vi "CSM - Broadcast Console.vi"() -> ()   [LabVIEW 2017]
doc: "CSM Debug Console, you can use this tool:\n\n1. Select an existing CSM instance, open the front panel and block diagram.\n2. Scan the API interfaces of existing CSM instances.\n3. Select an API interface, call synchronously or asynchronously, view the return value.\n4. View the overall program's running log."
uses:
  _Support/Typedef/_CSM_List Module Scope.ctl
  _Support/Typedef/_CSM_GlobalLog_MSG.ctl
  _Support/Typedef/_CSM_Response Source Message.ctl
  _Support/Typedef/_CSM_GlobalLog_MSG_TYPE.ctl
  _jksm/_action.ctl
  1437127e-efa5-494e-aa43-da9d647a7a6f.vi
  6c6a0a0d-4e90-432b-9646-7a8ac0ceadb8.vi
  <vilib>/addons/_JKI Toolkits/State Machine/_JKI_lib_State_Machine.llb/Parse State Queue__JKI_lib_State_Machine.vi
  AdvanceAPI/CSM - Convert Error to Argument.vi
  _Support/GlobalEvent/GEvt-Generate with Rule Check.vi
  AdvanceAPI/CSM - Keywords.vi
  _Support/GlobalEvent/Cache-GEvt Refs.vi
  _Support/GlobalEvent/LogFilter/LogFilter - Check.vi
  <vilib>/Utility/Data Type/Get Type Information.vi
  _csmHelper/lvcsmFile/lvcsm File Path.vi
  <vilib>/Utility/config.llb/Open Config Data.vi
  <vilib>/Utility/config.llb/Read Key.vi
  <vilib>/Utility/config.llb/Read Key (Boolean).vi
  <vilib>/Utility/config.llb/Read Key (String).vi
  <vilib>/Utility/Data Type/Get Array Information.vi
  <vilib>/Utility/config.llb/Get Key Names.vi
  _csmHelper/lvcsmFile/Path to lvcsm String.vi
  _csmHelper/lvcsmFile/lvcsm String to Path.vi
  <vilib>/Utility/config.llb/Read Key (I32).vi
  <vilib>/Utility/config.llb/Read Key (Double).vi
  <vilib>/Utility/config.llb/Close Config Data.vi
  _csmHelper/lvcsmFile/_Array of VData to VCluster.vi
  <vilib>/Utility/config.llb/Write Key.vi
  <vilib>/Utility/config.llb/Write Key (Boolean).vi
  <vilib>/Utility/config.llb/Remove Key.vi
  <vilib>/Utility/config.llb/Write Key (String).vi
  <vilib>/Utility/config.llb/Write Key (I32).vi
  <vilib>/Utility/config.llb/Write Key (Double).vi
  _Polymophic/Build Synchronous Message with Arguments.vi
  _Polymophic/Build No-Reply Asynchronous Message with Arguments.vi
  _Polymophic/Build Interrupt Broadcast Message.vi
  _Support/GlobalEvent/LogFilter/LogFilter.lvclass
  Communicable State Machine.lvlib
  _csmHelper/API with lvcsm Support/CSM-Helper API with lvcsm Support.lvlib
  _csmHelper/CSM-Helper.lvclass
  _Shared/CSM Shared.lvlib
  _ui/csm-ui-support.lvlib
  _jksm/_jkism_magic.lvlib
panel:
  in  "Scope":T1
  in  "Refresh CSMs Button":bool
  in  "CSM":string(combo)
  in  "Interface-Filter":enum16{"API-Only", "UserDef States", "All"}(ring)
  in  "Refresh API":bool
  in  "MsgString":string(combo)
  in  "Tab(Msg/Status)":enum32{"Message", "Status"}(tab)
  in  "Sync (-@)":bool
  in  "Async (->|)":bool
  in  "Timeout(s)":i32=10 caption="(s)" min=1 max=180 step=1 format="%.0p"
  in  "Broadcast":bool
  in  "Arguments":string
  in  "Revert Safe String":bool=TRUE
  out "Response":string
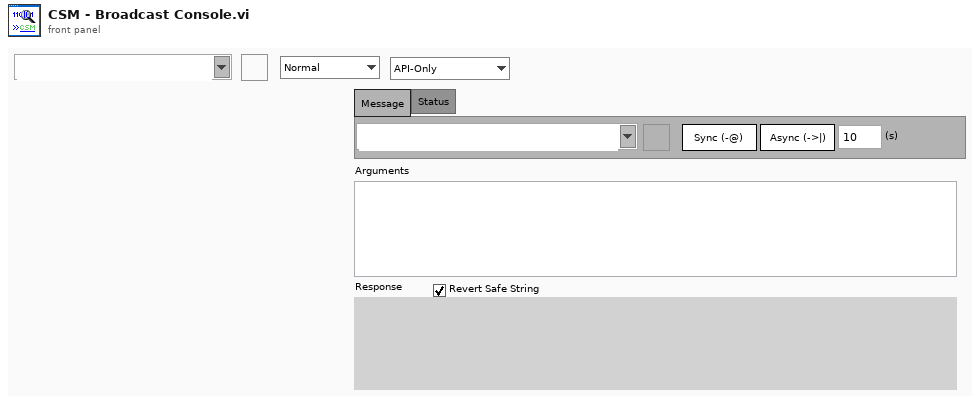
[diagram p1: front panel]
types:
  T1 = typedef "Communicable State Machine.lvlib/_CSM_List Module Scope.ctl" = enum16{"Normal", "System Only", "All"}
  T2 = enum32{"Invalid", "Standard", "Closed", "Hidden", "Minimized", "Maximized"}
  T3 = enum32{"invalid app kind", "Development System", "Run Time System", "Student Edition", "Embedded LabVIEW", "Evaluation", "Custom"}
  T4 = cluster{"Response Timeout(s)":i32, "History Length":i32, "History":string[], "Periodic Enable":bool, "Periodic threashold(#/s)":dbl, "Periodic Check Peroid(s)":dbl}
  T5 = typedef "_jkism_magic.lvlib/_action.ctl" = enum16{"Obtain", "Destroy", "Broadcast", "Post"}
  T6 = enum8{"Enabled", "Disabled", "Disabled and Grayed Out"}
  T7 = cluster{"Shift":bool, "Ctrl":bool, "Alt":bool, "Cmd":bool, "Opt":bool}
  T8 = cluster{"Core":cluster{"Current VI Reference":refnum<vi>, "Close Panel on Exit?":bool}, "CSM Global Log Event":refnum<user-event>, "MessageList":string[], "Toobar.advance":refnum<vi>[], "CSM Check History":string[], "History Length":i32}
  T9 = cluster{"Current VI Reference":refnum<vi>, "Close Panel on Exit?":bool}
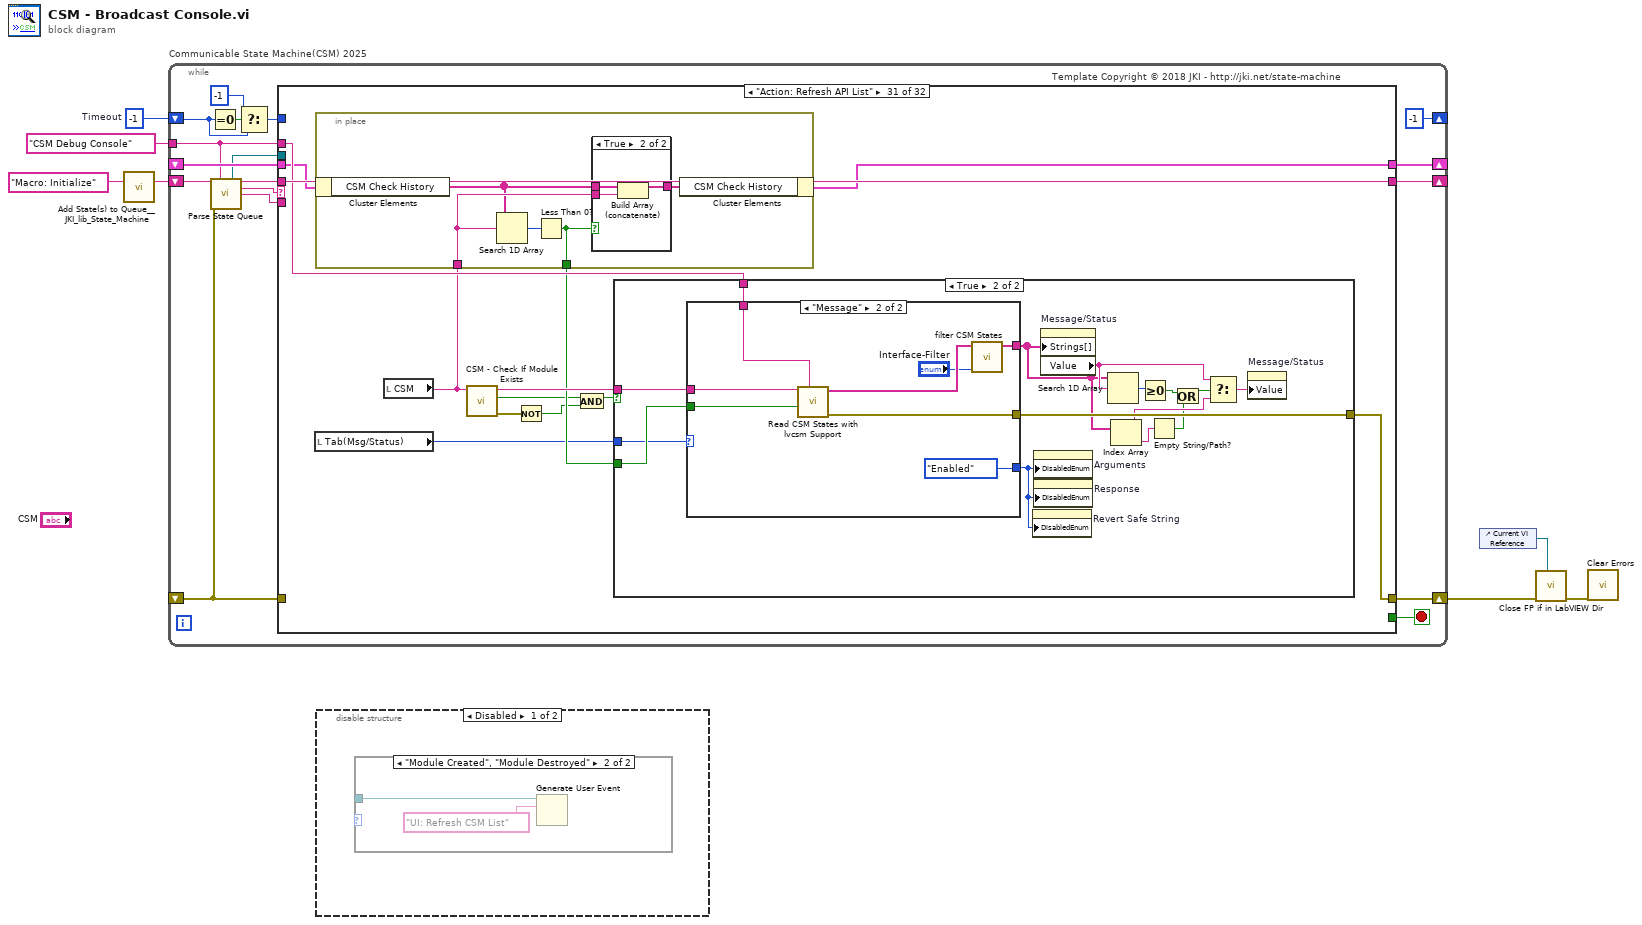
[diagram p0: block diagram]
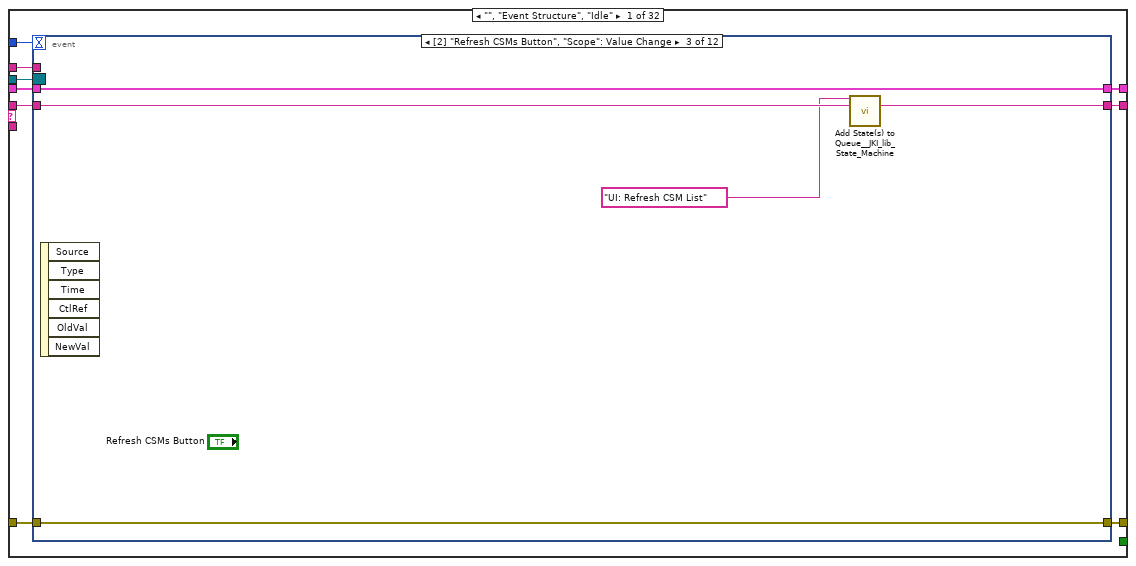
[diagram p4: hidden frame]
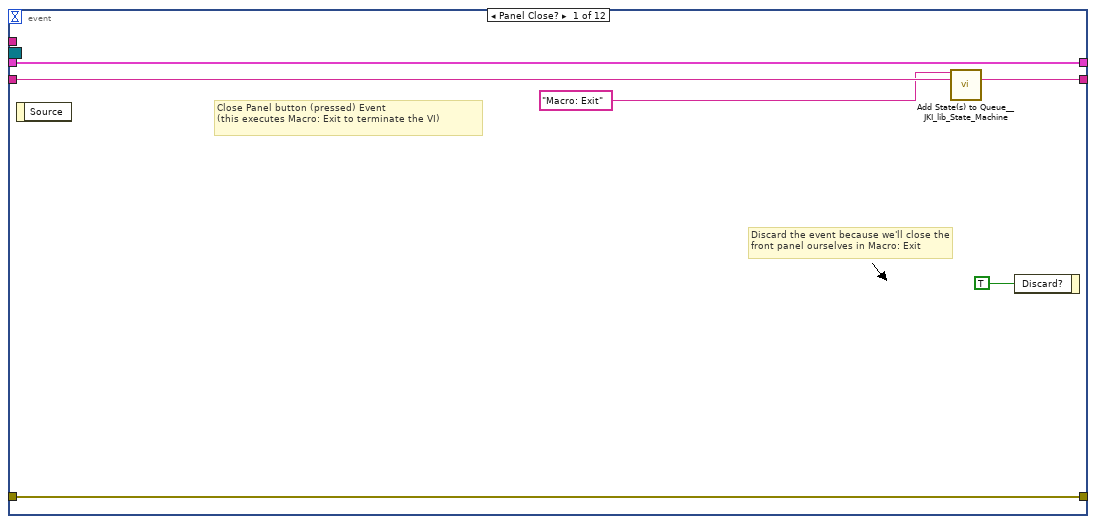
[diagram p5: hidden frame]
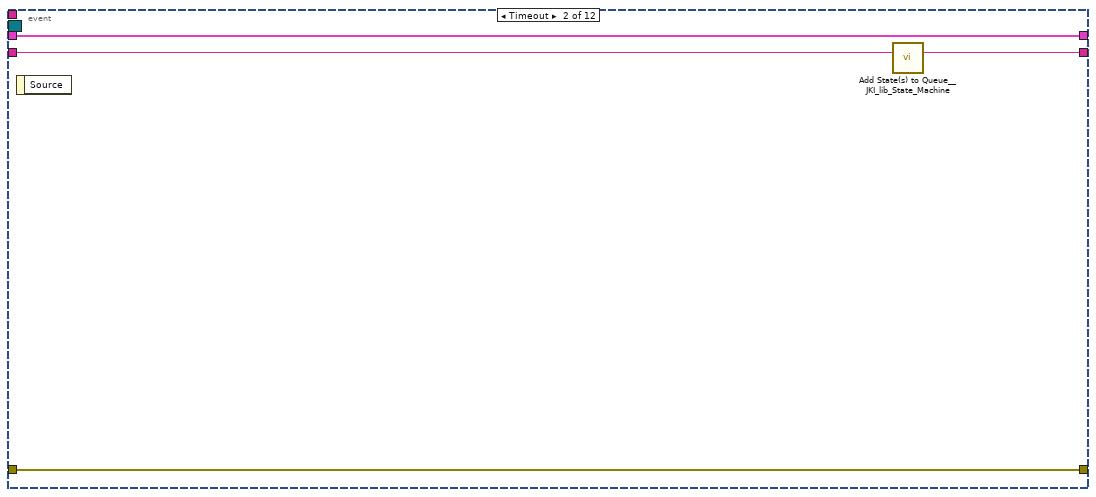
[diagram p6: hidden frame]
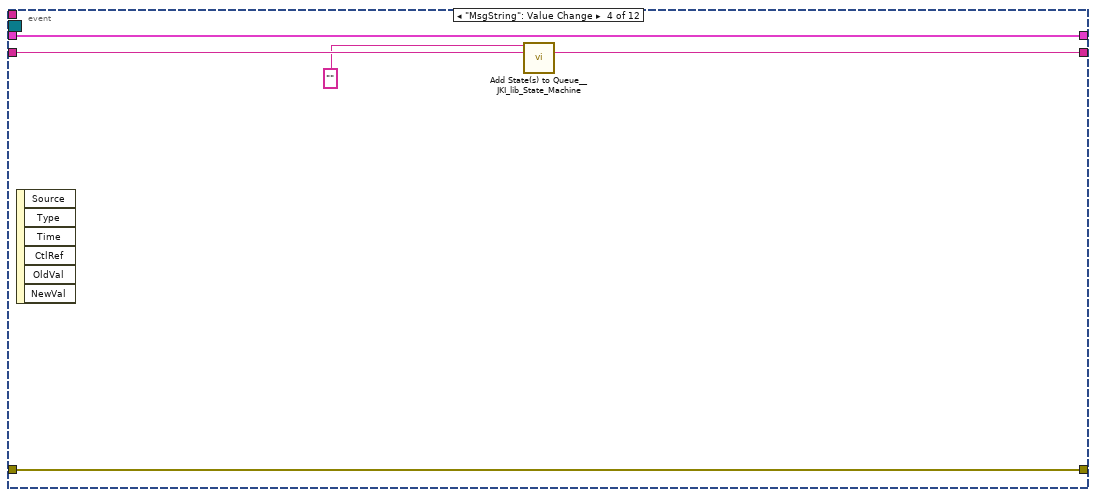
[diagram p7: hidden frame]
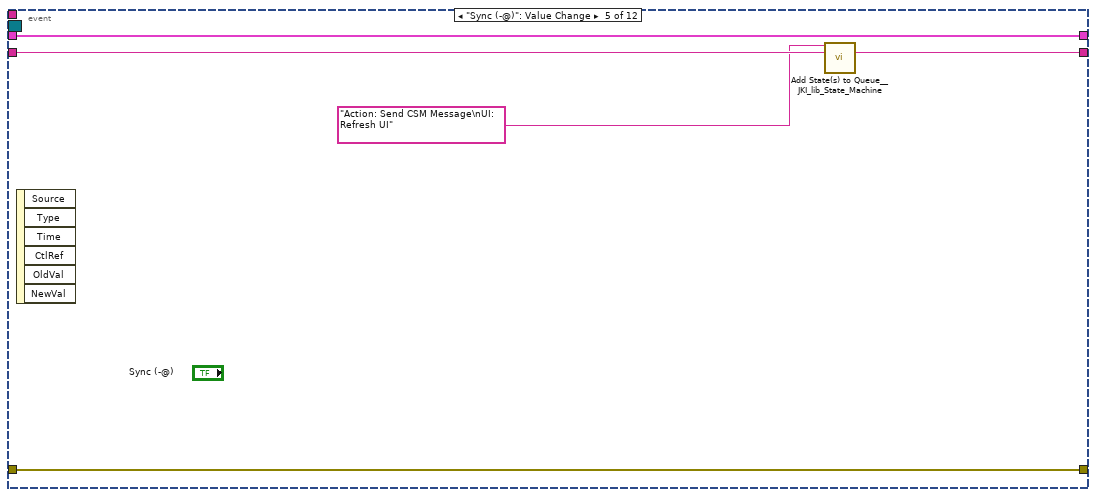
[diagram p8: hidden frame]
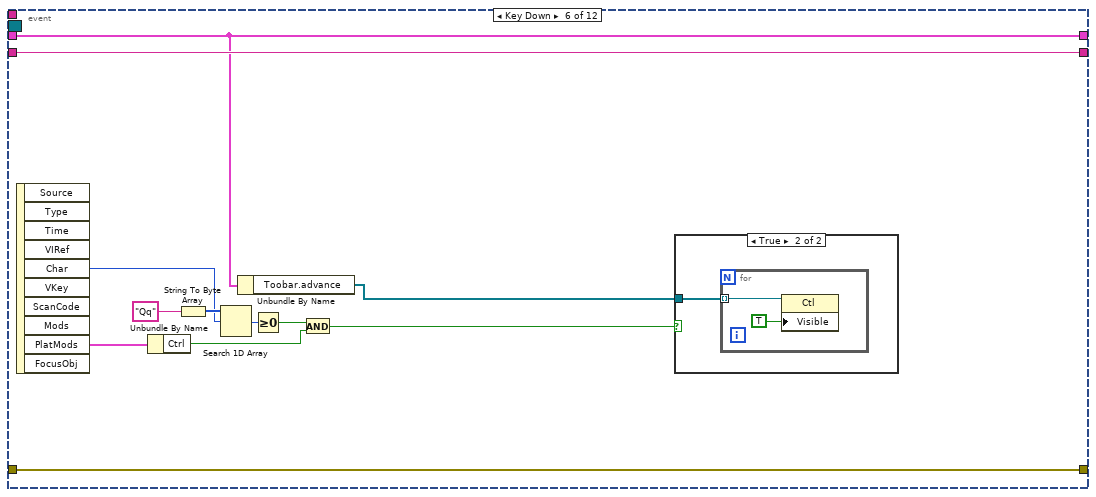
[diagram p9: hidden frame]
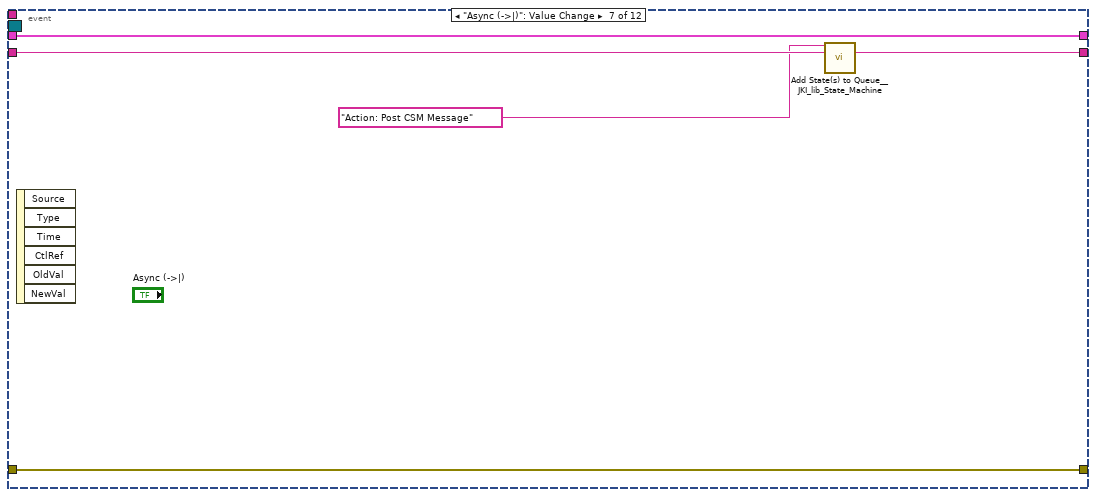
[diagram p11: hidden frame]
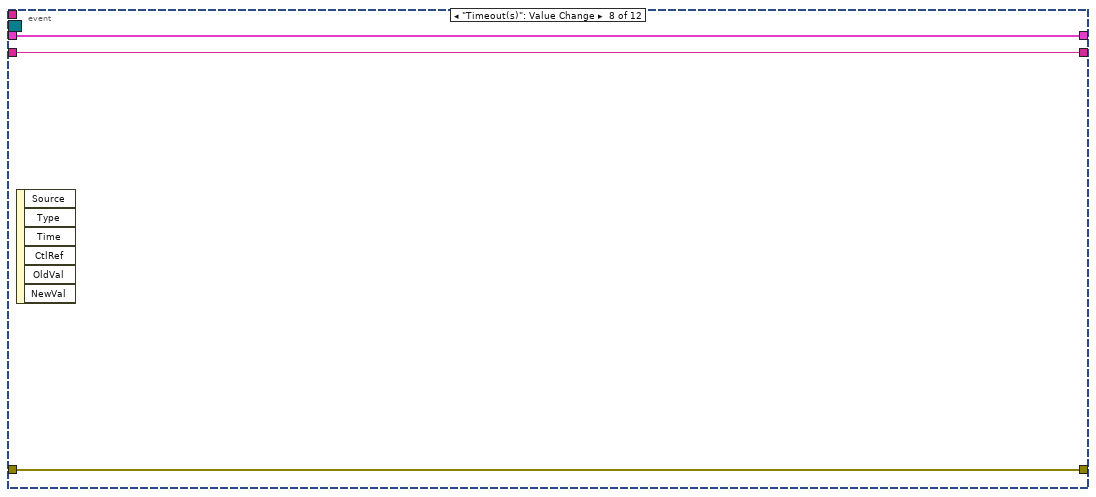
[diagram p12: hidden frame]
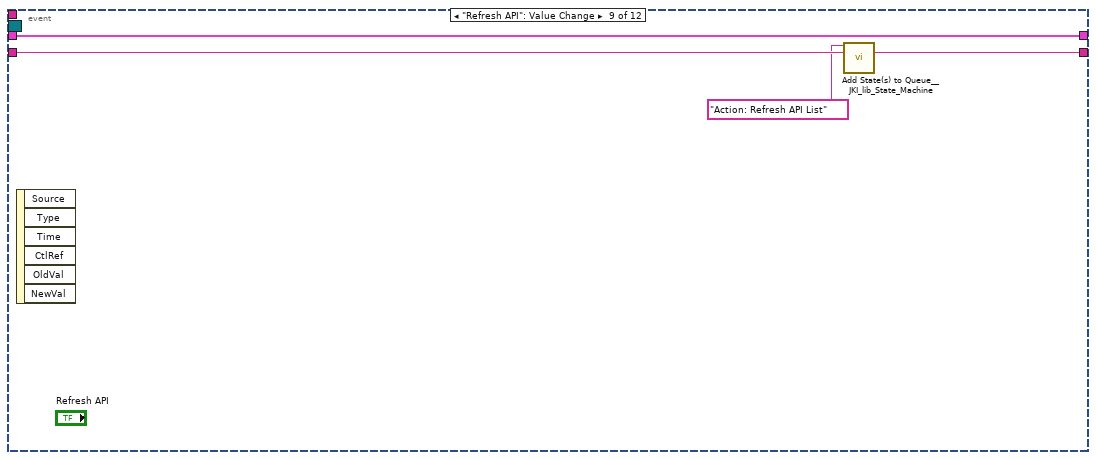
[diagram p13: hidden frame]
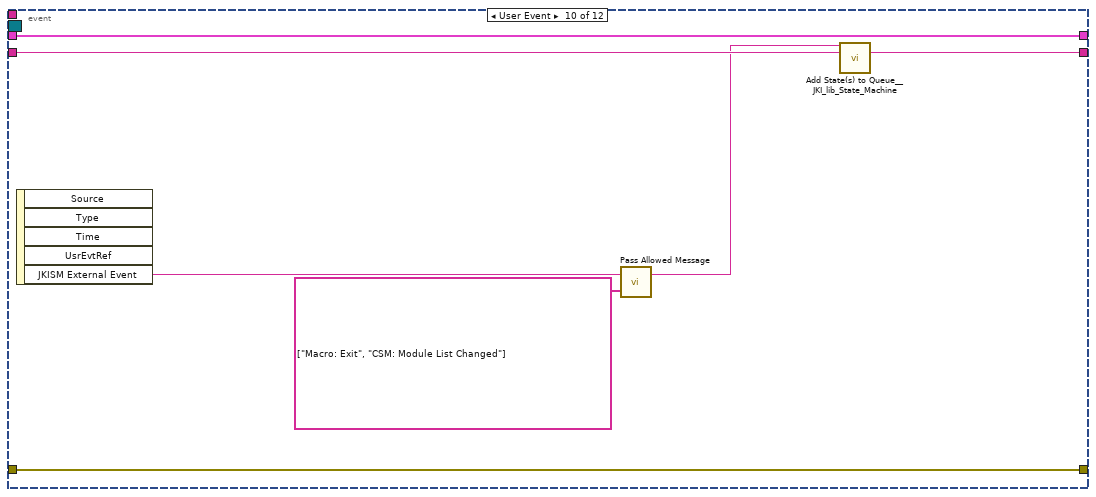
[diagram p14: hidden frame]
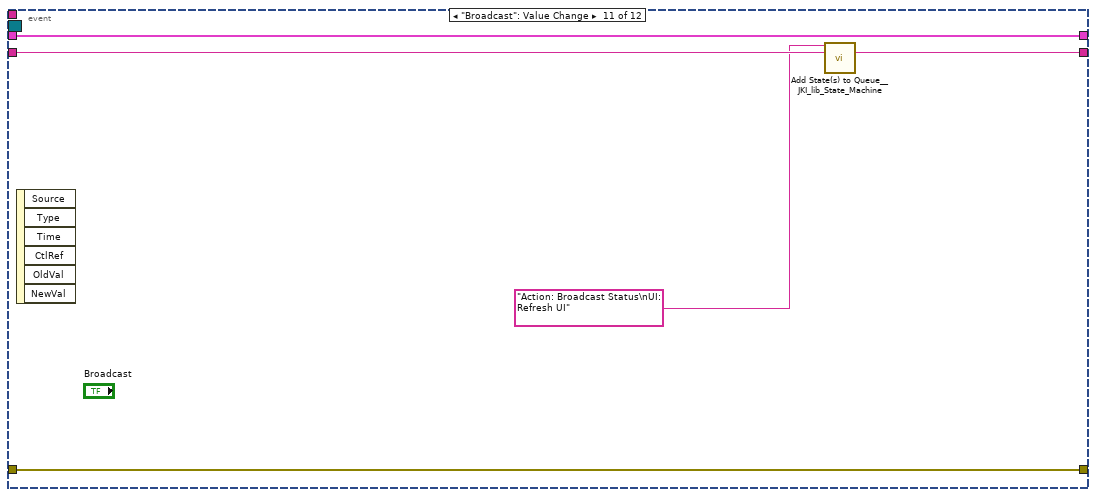
[diagram p15: hidden frame]
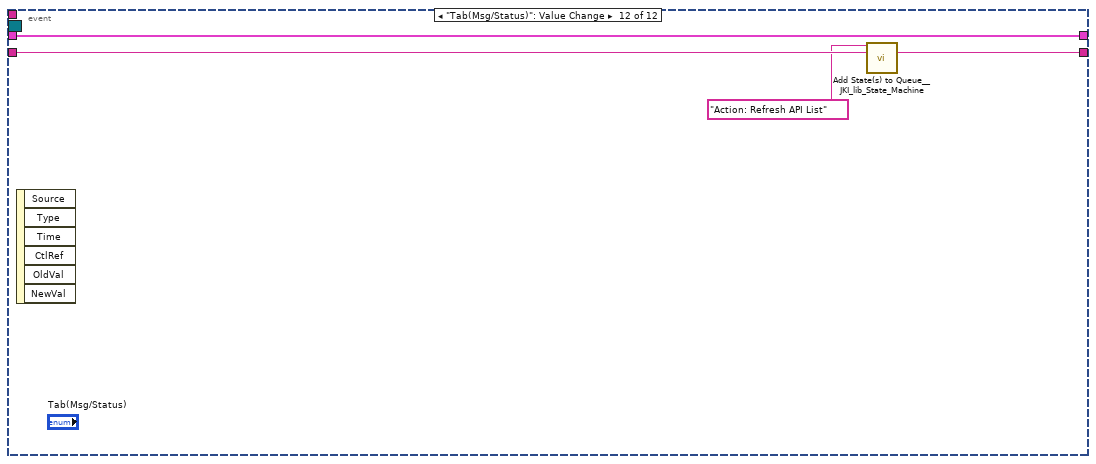
[diagram p16: hidden frame]
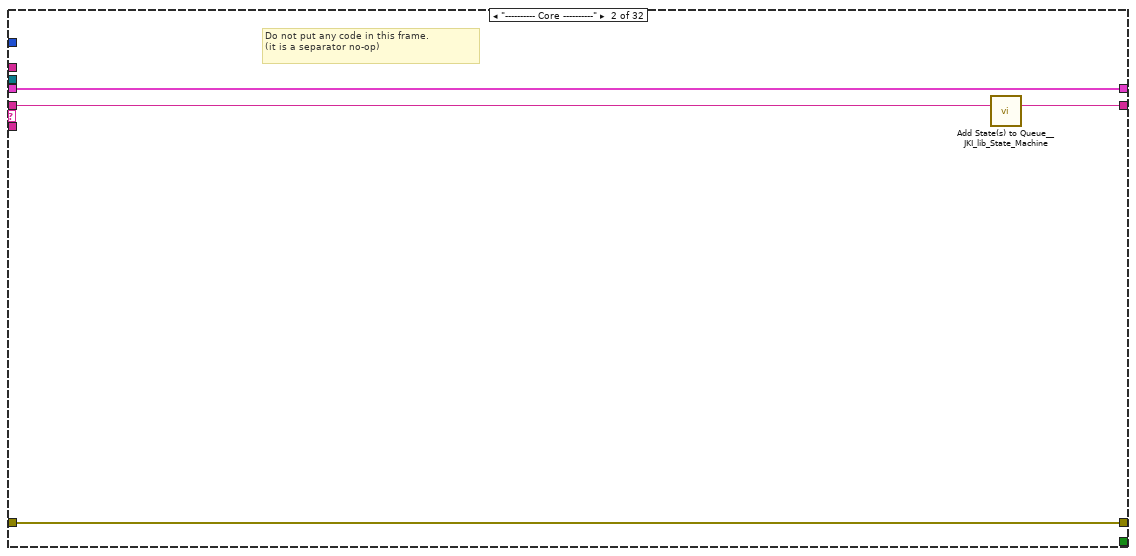
[diagram p17: hidden frame]
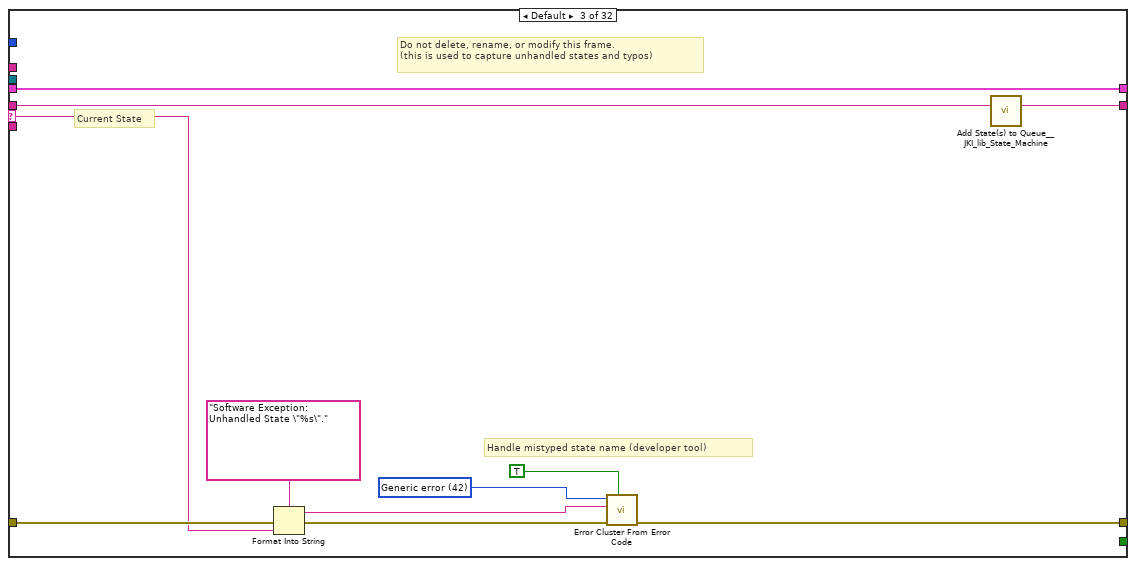
[diagram p18: hidden frame]
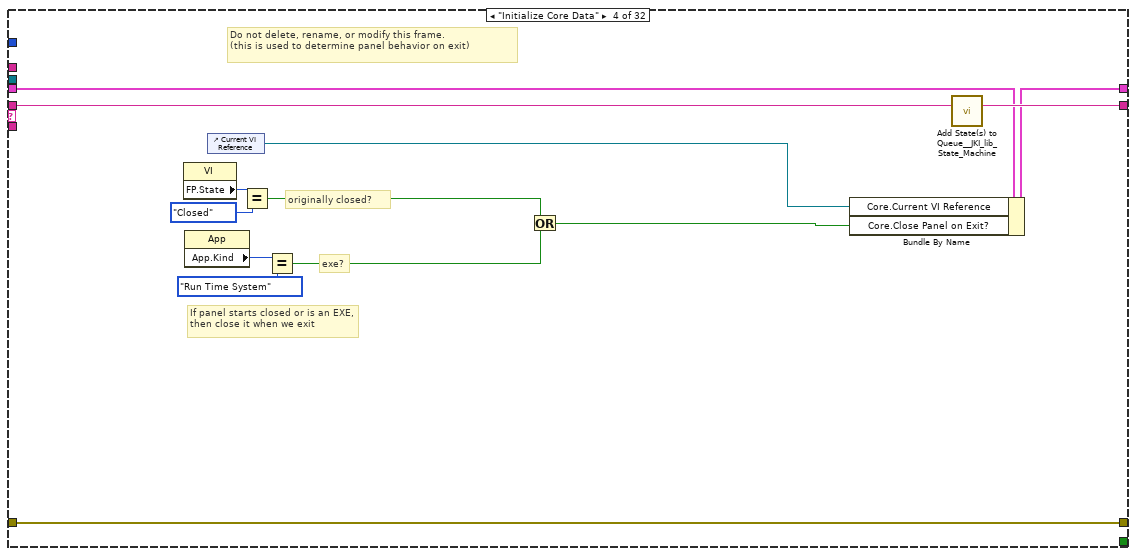
[diagram p19: hidden frame]
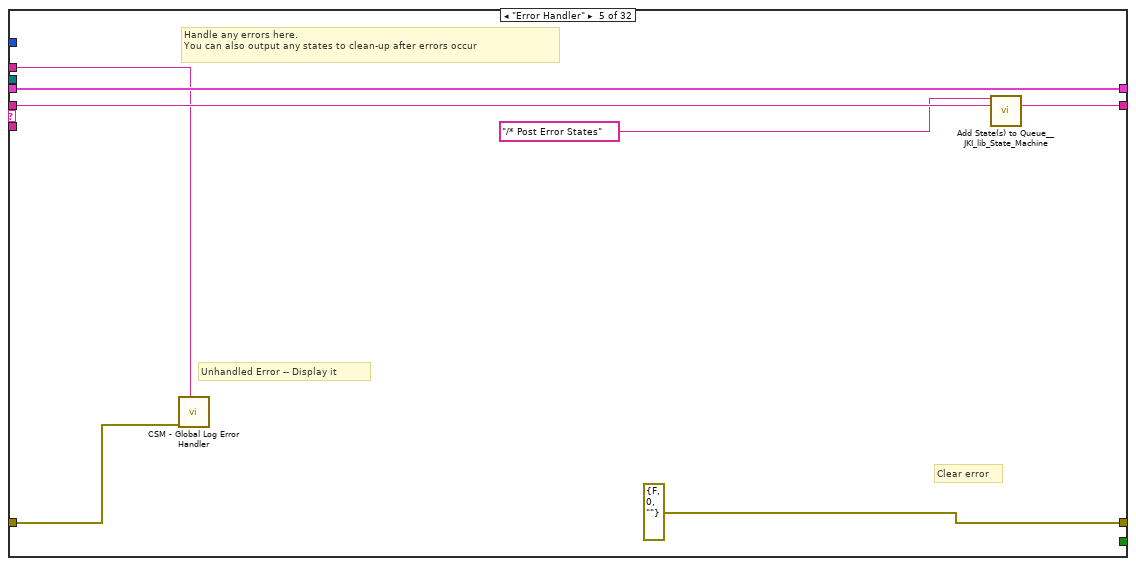
[diagram p20: hidden frame]
diagram:
  w5 = -1  # Timeout
  n1 = call <vilib>:"Add State(s) to Queue__JKI_lib_State_Machine.vi"("State(s) in (\"\")"="Macro: Initialize") -> ("States Out"=w6:string)  [unwired: 14 in]
  n2 = while "Communicable State Machine(CSM) 2025" {
    shift-right: [w17] -> _
    shift-left: _ -> [w16]
    shift-right: [w20] -> w2
    shift-left: _ -> [w15]
    shift-right: [w19] -> _
    shift-left: w6 -> [w21]
    tunnel: "CSM Debug Console" -> [w9]
    shift-right: [-1 ("Timeout")] -> _
    shift-left: w5 -> [w12]
    stop <- w18 stop-if-true
    # "Template Copyright © 2018 JKI - http://jki.net/state-machine"
    n3 = Equal To 0?(x=w12) -> (x = 0?=w14:bool)
    n4 = call "Parse State Queue.vi"("State Queue"=w21, "Current Module(\"\" to generate an ID)"=w9, "Error In (no error)"=w15) -> ("Event Registration Refnum"=w8:refnum<event-registration>, "Remaining States"=w23:string, "Current State"=w24:string, "Arguments"=w22:string)  [unwired: 9 in]
    n5 = Select(t=-1 ("Timeout"), s=w14, f=w12) -> (s? t:f=w11:i32)
    n6 = case shown="\"Action: Refresh API List\"" w24 {
      selector: w24 -> [_ _ w106 _ _ _ _ _ _ _ _ _ _ _ _ _ _ _ _ _ _ _ _ _ _ _ _ _ _ _ _ _]
      tunnel: w23 -> [w33 w105 w110 w129 w136 w141 w145 w155 w157 w167 w176 w188 w203 w207 w211 w219 w228 w239 w318 w329 w342 w345 w350 w355 w363 w367 w378 w404 w423 w437 w451 w502]
      tunnel: w22 -> [_ _ _ _ _ _ _ _ _ _ _ w184 _ _ _ _ w223 w233 w317 _ _ _ _ _ _ _ _ _ _ _ _ _]
      tunnel: w16 -> [w31 w102 w108 w122 w133 w139 w142 _ w156 w165 w175 w186 w198 w204 w208 w216 w226 w235 w315 w328 w341 w344 w347 w352 w360 w364 w376 w402 w421 w436 w446 w501]
      tunnel: [w30 w103 w112 w126 errorcluster {"status"=FALSE, "code"=0, "source"=""} ("error out") w138 w143 w152 w158 _ w170 w187 w199 w205 w209 w217 w224 w236 w319 w330 w343 w346 w348 w353 w361 w365 w373 w401 w420 w438 w448 w503] -> w20
      tunnel: w15 -> [w29 w103 w111 w126 w132 w138 w143 w152 w158 _ _ w187 w200 w205 w209 w217 w225 w237 w319 w330 w343 w346 w348 w353 w361 w365 _ _ _ w438 _ w503]
      tunnel: [w32 w104 w109 w128 w135 w140 w144 w154 w157 w167 w176 w188 w202 w206 w210 w218 w227 w238 w318 w329 w342 w345 w349 w354 w362 w366 w377 w403 w422 w437 w451 w502] -> w19
      tunnel: [_ _ _ _ _ TRUE _ _ _ _ _ _ _ _ _ _ _ _ _ _ _ _ _ _ _ _ _ _ _ _ _ _] -> w18
      tunnel: [w28 w102 w108 w127 w133 w139 w142 w153 w156 w166 w175 w180 w198 w204 w208 w216 w226 w235 w315 w328 w341 w344 w347 w352 w360 w364 w376 w402 w421 w436 w445 w501] -> w17
      tunnel: w11 -> [w27 _ _ _ _ _ _ _ _ _ _ _ _ _ _ _ _ _ _ _ _ _ _ _ _ _ _ _ _ _ _ _]
      tunnel: w9 -> [w26 _ _ _ w130 _ _ _ _ w162 w171 _ _ _ _ _ _ _ _ _ _ _ _ _ _ _ _ _ _ _ w449 w499]
      tunnel: w8 -> [w25 _ _ _ _ _ _ _ _ _ _ _ _ _ _ _ _ _ _ _ _ _ _ _ _ _ _ _ _ _ _ _]
      frame "", "Event Structure", "Idle" {
        n7 = event shown="[2] \"Refresh CSMs Button\", \"Scope\": Value Change" {
          selector: w25 -> [_ _ _ _ _ _ _ _ _ _ _ _]
          dyn-events: _ -> [_ _ _ _ _ _ _ _ _ _ _ _]
          timeout: w27 -> [_ _ _ _ _ _ _ _ _ _ _ _]
          tunnel: w33 -> [w39 w43 w46 w50 w55 w70 w75 w81 w83 w89 w94 w99]
          tunnel: [w38 w42 w45 w51 w56 w70 w76 w81 w84 w90 w95 w100] -> w32
          tunnel: w31 -> [w36 w40 w47 w52 w57 w59 w77 w79 w85 w91 w96 w101]
          tunnel: [w37 w41 w48 w53 w58 w69 w78 w80 _ w92 w97 _] -> w30
          tunnel: w29 -> [w37 w41 w48 w53 w58 w69 w78 w80 _ w92 w97 _]
          tunnel: [w36 w40 w47 w52 w57 w59 w77 w79 w85 w91 w96 w101] -> w28
          tunnel: w26 -> [_ _ _ _ _ _ _ _ _ _ _ _]
          event Panel Close? {
            # "Discard the event because we'll close the front panel ourselves in Macro: Exit"
            # "Close Panel button (pressed) Event\n(this executes Macro: Exit to terminate the VI)"
            n8 = event-data() -> ()  [unwired: 1 in, 1 out]
            n9 = call <vilib>:"Add State(s) to Queue__JKI_lib_State_Machine.vi"("State(s) in Front (\"\")"="Macro: Exit", "State(s) in (\"\")"=w39) -> ("States Out"=w38:string)  [unwired: 13 in]
            n10 = event-data("Discard?"=TRUE) -> ()  [unwired: 1 in, 1 out]
          }
          event Timeout {
            n11 = event-data() -> ()  [unwired: 1 in, 1 out]
            n12 = call <vilib>:"Add State(s) to Queue__JKI_lib_State_Machine.vi"("State(s) in (\"\")"=w43) -> ("States Out"=w42:string)  [unwired: 14 in]
          }
          event "Refresh CSMs Button": Value Change {
            n13 = event-data() -> ()  [unwired: 1 in, 6 out]
            n14 = call <vilib>:"Add State(s) to Queue__JKI_lib_State_Machine.vi"("State(s) in Front (\"\")"="UI: Refresh CSM List" ("State(s) in Front (\"\")"), "State(s) in (\"\")"=w46) -> ("States Out"=w45:string)  [unwired: 13 in]
          }
          event "MsgString": Value Change {
            n15 = event-data() -> ()  [unwired: 1 in, 6 out]
            n16 = call <vilib>:"Add State(s) to Queue__JKI_lib_State_Machine.vi"("State(s) in Front (\"\")"="" ("State(s) in Front (\"\")"), "State(s) in (\"\")"=w50) -> ("States Out"=w51:string)  [unwired: 13 in]
          }
          event "Sync (-@)": Value Change {
            n17 = event-data() -> ()  [unwired: 1 in, 6 out]
            n18 = call <vilib>:"Add State(s) to Queue__JKI_lib_State_Machine.vi"("State(s) in Front (\"\")"="Action: Send CSM Message\nUI: Refresh UI" ("State(s) in Front (\"\")"), "State(s) in (\"\")"=w55) -> ("States Out"=w56:string)  [unwired: 13 in]
          }
          event Key Down {
            n19 = event-data() -> ("Char"=w60:i16, "PlatMods"=w61:T7)  [unwired: 1 in, 8 out]
            n20 = Unbundle By Name(w61) -> ("Ctrl"=w64:bool)
            n21 = String To Byte Array(string="Qq") -> (unsigned byte array=w66:u8[])
            n22 = Search 1D Array(1D array=w66, element=w60) -> (index of element=w67:i32)  [unwired: 1 in]
            n23 = Unbundle By Name(w59) -> ("Toobar.advance"=w62:refnum<vi>[])
            n24 = Greater Or Equal To 0?(x=w67) -> (x >= 0?=w68:bool)
            n25 = And(x=w68, y=w64) -> (x .and. y?=w63:bool)
            n26 = case shown="True" w63 {
              tunnel: w62 -> [_ w71]
              frame False {
              }
              frame True {
                n27 = for {
                  tunnel: w71 -> [w73] mode=indexing
                  n28 = property class="Ctl"(reference=w73, "Visible"=TRUE) -> ()  [unwired: 1 in, 2 out]
                }
              }
            }
          }
          event "Async (->|)": Value Change {
            n29 = event-data() -> ()  [unwired: 1 in, 6 out]
            n30 = call <vilib>:"Add State(s) to Queue__JKI_lib_State_Machine.vi"("State(s) in Front (\"\")"="Action: Post CSM Message" ("State(s) in Front (\"\")"), "State(s) in (\"\")"=w75) -> ("States Out"=w76:string)  [unwired: 13 in]
          }
          event "Timeout(s)": Value Change {
            n31 = event-data() -> ()  [unwired: 1 in, 6 out]
          }
          event "Refresh API": Value Change {
            n32 = event-data() -> ()  [unwired: 1 in, 6 out]
            n33 = call <vilib>:"Add State(s) to Queue__JKI_lib_State_Machine.vi"("State(s) in Front (\"\")"="Action: Refresh API List" ("State(s) in Front (\"\")"), "State(s) in (\"\")"=w83) -> ("States Out"=w84:string)  [unwired: 13 in]
          }
          event User Event {
            n34 = event-data() -> ("JKISM External Event"=w88:string)  [unwired: 1 in, 4 out]
            n35 = call "Pass Allowed Message.vi"("Allowed Message"=string[] ["Macro: Exit", "CSM: Module List Changed"], "JKISM External Event"=w88) -> ("States"=w87:string)  [unwired: 1 in]
            n36 = call <vilib>:"Add State(s) to Queue__JKI_lib_State_Machine.vi"("State(s) in Front (\"\")"=w87, "State(s) in (\"\")"=w89) -> ("States Out"=w90:string)  [unwired: 13 in]
          }
          event "Broadcast": Value Change {
            n37 = event-data() -> ()  [unwired: 1 in, 6 out]
            n38 = call <vilib>:"Add State(s) to Queue__JKI_lib_State_Machine.vi"("State(s) in Front (\"\")"="Action: Broadcast Status\nUI: Refresh UI" ("State(s) in Front (\"\")"), "State(s) in (\"\")"=w94) -> ("States Out"=w95:string)  [unwired: 13 in]
          }
          event "Tab(Msg/Status)": Value Change {
            n39 = event-data() -> ()  [unwired: 1 in, 6 out]
            n40 = call <vilib>:"Add State(s) to Queue__JKI_lib_State_Machine.vi"("State(s) in Front (\"\")"="Action: Refresh API List" ("State(s) in Front (\"\")"), "State(s) in (\"\")"=w99) -> ("States Out"=w100:string)  [unwired: 13 in]
          }
        }
      }
      frame "---------- Core ----------" {
        # "Do not put any code in this frame.\n(it is a separator no-op)"
        n41 = call <vilib>:"Add State(s) to Queue__JKI_lib_State_Machine.vi"("State(s) in (\"\")"=w105) -> ("States Out"=w104:string)  [unwired: 14 in]
      }
      frame Default {
        w115 = 42 items=["No error", "Argument error", "Memory is full", "Out of zone", "End of file", "File already open", "Generic file I/O error", "File not found", "File permission error", "Disk is full", "Duplicate path", "Too many files open", "System feature not enabled", "Resource file not found", "Cannot add resource", "Resource not found", "Image not found", "Image memory error", "Pen does not exist", "Config type invalid", "Config token not found", "Config parse error", "Config memory error", "Bad external code format", "Bad external code offset", "External code not present", "Null window", "Destroy window error", "Null menu", "Print aborted", "Bad print record", "Print driver error", "Windows error during printing", "Memory error during printing", "Print dialog error", "Generic print error", "Invalid device refnum", "Device not found", "Device parameter error", "Device unit error", "Cannot open device", "Device call aborted", "Generic error", "Cancelled by user", "Object ID too low", "Object ID too high", "Object not in heap", "Unknown heap", "Unknown object (invalid DefProc)", "Unknown object (DefProc not in table)", "Message out of range", "Invalid (null) method", "Unknown message", "Manager call not supported", "Bad address", "Network operation in progress", "Network operation timed out", "Connection is busy", "Network attribute not supported", "Network error", "Address in use", "System out of memory", "Connection aborted", "Connection refused", "Not connected", "Already connected", "Connection closed", "Initialization error (interapplication manager)", "Bad occurrence", "Wait on unbound occurrence handler", "Occurrence queue overflow", "Datalog type conflict", "Unused", "Unrecognized type (interapplication manager)", "Memory corrupt", "Failed to make temporary DLL", "Old CIN version", "Drag socket not found", "Failed to load drop-object", "Failed to register OLE object", "Failed to release OLE object", "Format specifier type mismatch", "Unknown format specifier", "Too few format specifiers", "Too many format specifiers", "Scan failed", "Newer CIN version", "Error converting to variant", "Runtime menu error", "Password tampered", "Variant attribute not found", "Incompatible variant data type", "Event data is not available", "Event Store is not present", "Occurrence is not found", "Event Queue is not created", "Event info is not available", "Refnum passed is NULL", "Error retrieving Class GUID", "Error retrieving CoClass GUID", "Error retrieving TypeLib GUID.", "Bad built application magic bytes.", "Specific driver is different from the specific driver associated with the Logical Name.", "There is no session opened to the class driver.", "Max Error", "MAX - Error with config objects", "MAX - Error loading configuration", "MAX - Group not supported"]
        # "Current State"
        # "Do not delete, rename, or modify this frame.\n(this is used to capture unhandled states and typos)"
        # "Handle mistyped state name (developer tool)"
        n42 = Format Into String(format string="Software Exception: Unhandled State \"%s\"." ("message"), error in=w111, w106) -> (resulting string=w114:string, error out=w113:errorcluster)  [unwired: 1 in]
        n43 = call <vilib>:"Error Cluster From Error Code.vi"("show call chain? (False)"=TRUE, "error in (no error)"=w113, "error message (\"\")"=w114, "error code (0)"=w115) -> ("error out"=w112:errorcluster)  [unwired: 5 in]
        n44 = call <vilib>:"Add State(s) to Queue__JKI_lib_State_Machine.vi"("State(s) in (\"\")"=w110) -> ("States Out"=w109:string)  [unwired: 14 in]
      }
      frame "Initialize Core Data" {
        # "Do not delete, rename, or modify this frame.\n(this is used to determine panel behavior on exit)"
        # "originally closed?"
        # "exe?"
        # "If panel starts closed or is an EXE, then close it when we exit"
        n45 = property class="VI"() -> ("FP.State"=w119:T2)  [unwired: 2 in, 2 out]
        n46 = property class="App"() -> ("App.Kind"=w125:T3)  [unwired: 2 in, 2 out]
        n47 = control-ref of="Current VI Reference"() -> (w120:refnum<vi>)
        n48 = Equal?(x=w119, y=T2."Closed" ("Front Panel Window:State")) -> (x = y?=w117:bool)
        n49 = Equal?(x=w125, y=T3."Run Time System" ("Application:Kind")) -> (x = y?=w123:bool)
        n50 = Or(x=w117, y=w123) -> (x .or. y?=w121:bool)
        n51 = Bundle By Name(cluster=w122, "Core.Current VI Reference"=w120, "Core.Close Panel on Exit?"=w121) -> (w127:T8)
        n52 = call <vilib>:"Add State(s) to Queue__JKI_lib_State_Machine.vi"("State(s) in (\"\")"=w129) -> ("States Out"=w128:string)  [unwired: 14 in]
      }
      frame "Error Handler" {
        # "Unhandled Error -- Display it"
        # "Handle any errors here.\nYou can also output any states to clean-up after errors occur"
        # "Clear error"
        n53 = call "CSM - Global Log Error Handler.vi"("Place (\"\" to Use VI's Name)"=w130, "Error In"=w132) -> ()  [unwired: 9 in, 1 out]
        n54 = call <vilib>:"Add State(s) to Queue__JKI_lib_State_Machine.vi"("State(s) in Front (\"\")"="/* Post Error States", "State(s) in (\"\")"=w136) -> ("States Out"=w135:string)  [unwired: 13 in]
      }
      frame "Exit" {
        # "Do not put any code in this frame.\n(No errors that occur here will be handled.)"
        n55 = call <vilib>:"Add State(s) to Queue__JKI_lib_State_Machine.vi"("State(s) in (\"\")"=w141) -> ("States Out"=w140:string)  [unwired: 14 in]
      }
      frame "---------- Data ----------" {
        # "Do not put any code in this frame.\n(It is a separator no-op. You can make a copy of this frame to create a new Data frame)"
        n56 = call <vilib>:"Add State(s) to Queue__JKI_lib_State_Machine.vi"("State(s) in (\"\")"=w145) -> ("States Out"=w144:string)  [unwired: 14 in]
      }
      frame "Data: Initialize" {
        w146 = 50  # History Length
        w147 = string[] []  # CSM Check History
        w148 = refnum<vi>[] []  # Toobar.advance
        w149 = string[] []  # MessageList
        w150 = refnum<user-event> refnum  # CSM Global Log Event
        w151 = T9 {"Current VI Reference"=refnum, "Close Panel on Exit?"=FALSE}  # Core
        # "Initialize the shift-register data, here.\n(data names are defined by what you wire into the bundle function)"
        n57 = Bundle("Core"=w151, "CSM Global Log Event"=w150, "MessageList"=w149, "Toobar.advance"=w148, "CSM Check History"=w147, "History Length"=w146) -> (w153:T8)  [unwired: 1 in]
        n58 = call <vilib>:"Add State(s) to Queue__JKI_lib_State_Machine.vi"("State(s) in (\"\")"=w155) -> ("States Out"=w154:string)  [unwired: 14 in]
      }
      frame "Data: Initialize References" {
      }
      frame "Data: Load Arguments Config File" {
        n59 = call "lvcsm Read Cluster.vim"("Section"=w162, "Default Prototype"=T4 {"Response Timeout(s)"=30, "History Length"=50, "History"=[], "Periodic Enable"=TRUE, "Periodic threashold(#/s)"=0.5, "Periodic Check Peroid(s)"=3.0}) -> ("Cluster (Dup)"=w164:T4)  [unwired: 8 in, 1 out]
        n60 = Unbundle By Name(w164) -> ("Response Timeout(s)"=w163:i32, "History Length"=w159:i32, "History"=w161:string[])  [unwired: 3 out]
        n61 = local write "Timeout(s)"(w163) -> ()
        n62 = Bundle By Name(cluster=w165, "History Length"=w159, "MessageList"=w161) -> (w166:T8)
      }
      frame "Data: Save Arguments Config File" {
        n63 = Unbundle By Name(w175) -> ("MessageList"=w172:string[], "History Length"=w168:i32)
        n64 = local read "Timeout(s)"() -> (w173:i32)
        n65 = Bundle By Name(cluster=T4 {"Response Timeout(s)"=30, "History Length"=50, "History"=[], "Periodic Enable"=TRUE, "Periodic threashold(#/s)"=0.5, "Periodic Check Peroid(s)"=3.0}, "History"=w172, "Response Timeout(s)"=w173, "History Length"=w168) -> (w174:T4)
        n66 = call "lvcsm Write Cluster.vim"("Section"=w171, "Configuration"=w174) -> ("error out"=w170:errorcluster)  [unwired: 9 in]
      }
      frame "Data: Update Message List" {
        n67 = Unbundle By Name(w186) -> ("MessageList"=w185:string[], "History Length"=w177:i32)
        n68 = call "CSM - Revert Arguments-Safe String.vi"("Safe Argument String"=w184) -> ("Origin Argument String"=w183:string)  [unwired: 8 in]
        n69 = Build Array (concatenate)(w183, w185) -> (w182:string[])
        n70 = for {
          tunnel: w182 -> [w192] mode=indexing
          shift-right: [w191] -> w178
          shift-left: string[] [] -> [w190]
          i -> [w189]
          n71 = Search 1D Array(1D array=w190, element=w192) -> (index of element=w193:i32)  [unwired: 1 in]
          n72 = case shown="-1" w193 {
            tunnel: w192 -> [_ w197]
            tunnel: [w194 w195] -> w191
            tunnel: w190 -> [w194 w196]
            tunnel: w189 -> [_ _]
            frame Default {
            }
            frame -1 {
              n73 = Build Array (concatenate)(w196, w197) -> (w195:string[])
            }
          }
        }
        n74 = Array Subset(array=w178, length=w177) -> (w179:string[])  [unwired: 1 in]
        n75 = Bundle By Name(cluster=w186, "MessageList"=w179) -> (w180:T8)
      }
      frame "Data: Cleanup" {
        # "Cleanup any data and references, here.\n(this is called automatically, by the Macro: Exit)"
        n76 = Unbundle By Name(w198) -> ("Core.Current VI Reference"=w201:refnum<vi>)
        n77 = Close Reference(reference=w201, error in (no error)=w200) -> (error out=w199:errorcluster)
        n78 = call <vilib>:"Add State(s) to Queue__JKI_lib_State_Machine.vi"("State(s) in (\"\")"=w203) -> ("States Out"=w202:string)  [unwired: 14 in]
      }
      frame "---------- Events ----------" {
        # "Do not put any code in this frame.\n(It is a separator no-op. You can make a copy of this frame to create a new UI frame)"
        n79 = call <vilib>:"Add State(s) to Queue__JKI_lib_State_Machine.vi"("State(s) in (\"\")"=w207) -> ("States Out"=w206:string)  [unwired: 14 in]
      }
      frame "---------- UI ----------" {
        # "Do not put any code in this frame.\n(It is a separator no-op. You can make a copy of this frame to create a new UI frame)"
        n80 = call <vilib>:"Add State(s) to Queue__JKI_lib_State_Machine.vi"("State(s) in (\"\")"=w211) -> ("States Out"=w210:string)  [unwired: 14 in]
      }
      frame "UI: Initialize" {
        # "Initialize the User Interface, here.\n(this is called automatically, by the Macro: Init)"
        n81 = Unbundle By Name(w216) -> ("Toobar.advance"=w215:refnum<vi>[])
        n82 = disable-structure shown="Disabled" {
          disable-tunnel: w215 -> [w220 _]
          frame Disabled {
            n83 = for {
              tunnel: w220 -> [w222] mode=indexing
              n84 = property class="Ctl"(reference=w222, "Visible"=FALSE) -> ()  [unwired: 1 in, 2 out]
            }
          }
          frame Enabled {
          }
        }
        n85 = local write "Tab(Msg/Status)"(enum32{"Message", "Status"}."Message" ("Tab(Msg/Status)")) -> ()
        n86 = local write "Response"(" " ("State History")) -> ()
        n87 = local write "Interface-Filter"(enum16{"API-Only", "UserDef States", "All"}."UserDef States" ("Interface-Filter")) -> ()
        n88 = call <vilib>:"Add State(s) to Queue__JKI_lib_State_Machine.vi"("State(s) in (\"\")"=w219) -> ("States Out"=w218:string)  [unwired: 14 in]
      }
      frame "UI: Cursor Set" {
        # "Argument"
        # "Set and Unset Cursor Busy.\n(Usage: \"UI: Cursor Set >> Busy|Idle\")"
        n89 = case shown="\"Idle\", Default" w223 {
          tunnel: w225 -> [w230 w232]
          tunnel: [w229 w231] -> w224
          frame "Idle", Default {
            n90 = call <vilib>:"Unset Busy.vi"("error in (no error)"=w230) -> ("error out"=w229:errorcluster)  [unwired: 10 in]
          }
          frame "Busy" {
            n91 = call <vilib>:"Set Busy.vi"("error in (no error)"=w232) -> ("error out"=w231:errorcluster)  [unwired: 9 in, 1 out]
          }
        }
        n92 = call <vilib>:"Add State(s) to Queue__JKI_lib_State_Machine.vi"("State(s) in (\"\")"=w228) -> ("States Out"=w227:string)  [unwired: 14 in]
      }
      frame "UI: Front Panel State" {
        # "Argument"
        # "Set Front Panel Open or Closed\n(Usage: \"UI: Front Panel State >> Open|Close\")"
        n93 = Unbundle By Name(w235) -> ("Core.Current VI Reference"=w234:refnum<vi>)
        n94 = case shown="\"Minimize\", \"Minimized\"" w233 {
          tunnel: w237 -> [w245 w260 w271 w284 w297]
          tunnel: [w247 w261 w273 w286 w299] -> w236
          tunnel: w234 -> [w246 w258 w272 w285 w298]
          frame "Open", "Standard", Default {
            w240 = T2."Standard" ("State")
            n95 = property class="VI"(reference=w246, error in=w245) -> (reference out=w243:refnum<vi>, error out=w244:errorcluster, "FP.State"=w242:T2)
            n96 = Not Equal?(x=w242, y=w240) -> (x != y?=w241:bool)
            n97 = case shown="True" w241 {
              tunnel: [w251 w253] -> w247
              tunnel: w244 -> [w250 w253]
              tunnel: w243 -> [w249 _]
              tunnel: w240 -> [w248 _]
              frame True {
                n98 = invoke class="VI" method="FP.Open"(reference=w249, error in=w250, "Activate"=TRUE, "State"=w248) -> (error out=w251:errorcluster)  [unwired: 1 in, 4 out]
              }
              frame False {
              }
            }
          }
          frame "Close", "Closed" {
            n99 = property class="VI"(reference=w258, error in=w260) -> (reference out=w257:refnum<vi>, error out=w259:errorcluster, "FP.State"=w255:T2)
            n100 = Not Equal?(x=w255, y=T2."Closed" ("Front Panel Window:State")) -> (x != y?=w254:bool)
            n101 = case shown="True" w254 {
              tunnel: [w262 w265] -> w261
              tunnel: w259 -> [w262 w264]
              tunnel: w257 -> [_ w263]
              frame False {
              }
              frame True {
                n102 = invoke class="VI" method="FP.Close"(reference=w263, error in=w264) -> (error out=w265:errorcluster)  [unwired: 1 in, 2 out]
              }
            }
          }
          frame "Hidden", "Hide" {
            w266 = T2."Hidden" ("State")
            n103 = property class="VI"(reference=w272, error in=w271) -> (reference out=w269:refnum<vi>, error out=w270:errorcluster, "FP.State"=w268:T2)
            n104 = Not Equal?(x=w268, y=w266) -> (x != y?=w267:bool)
            n105 = case shown="True" w267 {
              tunnel: [w277 w278] -> w273
              tunnel: w270 -> [w276 w278]
              tunnel: w269 -> [w275 _]
              tunnel: w266 -> [w274 _]
              frame True {
                n106 = invoke class="VI" method="FP.Open"(reference=w275, error in=w276, "State"=w274) -> (error out=w277:errorcluster)  [unwired: 2 in, 4 out]
              }
              frame False {
              }
            }
          }
          frame "Minimize", "Minimized" {
            w279 = T2."Minimized" ("State")
            n107 = property class="VI"(reference=w285, error in=w284) -> (reference out=w282:refnum<vi>, error out=w283:errorcluster, "FP.State"=w281:T2)
            n108 = Not Equal?(x=w281, y=w279) -> (x != y?=w280:bool)
            n109 = case shown="True" w280 {
              tunnel: [w290 w291] -> w286
              tunnel: w283 -> [w289 w291]
              tunnel: w282 -> [w288 _]
              tunnel: w279 -> [w287 _]
              frame True {
                n110 = invoke class="VI" method="FP.Open"(reference=w288, error in=w289, "State"=w287) -> (error out=w290:errorcluster)  [unwired: 2 in, 4 out]
              }
              frame False {
              }
            }
          }
          frame "Maximize", "Maximized" {
            w292 = T2."Maximized" ("State")
            n111 = property class="VI"(reference=w298, error in=w297) -> (reference out=w295:refnum<vi>, error out=w296:errorcluster, "FP.State"=w294:T2)
            n112 = Not Equal?(x=w294, y=w292) -> (x != y?=w293:bool)
            n113 = case shown="True" w293 {
              tunnel: [w303 w304] -> w299
              tunnel: w296 -> [w302 w304]
              tunnel: w295 -> [w301 _]
              tunnel: w292 -> [w300 _]
              frame True {
                n114 = invoke class="VI" method="FP.Open"(reference=w301, error in=w302, "State"=w300) -> (error out=w303:errorcluster)  [unwired: 2 in, 4 out]
              }
              frame False {
              }
            }
          }
        }
        n115 = call <vilib>:"Add State(s) to Queue__JKI_lib_State_Machine.vi"("State(s) in (\"\")"=w239) -> ("States Out"=w238:string)  [unwired: 14 in]
      }
      frame "UI: Autoset Arguments" {
        n116 = call "CSM - Revert Arguments-Safe String.vi"("Safe Argument String"=w317) -> ("Origin Argument String"=w305:string)  [unwired: 8 in]
        n117 = control-ref of="CSM"() -> (w312:refnum<vi>)
        n118 = call "Remove Comments from Single-line.vi"("single-line text"=w305) -> ("single-line text without comments"=w316:string)  [unwired: 2 in]
        n119 = property on="Property Node" class="CmbBox"(reference=w312) -> (reference out=w310:refnum<vi>, "Strings[]"=w311:string[])  [unwired: 1 in, 1 out]
        n120 = call "Split Single-line Message.vi"("single-line text"=w316) -> ("state"=w314:string, "args"=w313:string, "source/target"=w307:string)  [unwired: 6 in, 1 out]
        n121 = case shown="\"<interrupt>\", \"<status>\"" w307 {
          selector: w307 -> [w320 _]
          tunnel: [w320 w322] -> w306
          tunnel: w305 -> [_ w323]
          frame Default {
            n122 = property on="Tab(Msg/Status)" class="TabCtl (strict)"("Val(Sgnl)"=enum32{"Message", "Status"}."Message" ("Tab(Msg/Status)")) -> ()  [unwired: 2 in, 2 out]
          }
          frame "<interrupt>", "<status>" {
            n123 = Match Pattern(string=w323, regular expression="//") -> (after substring=w322:string)  [unwired: 1 in, 3 out]
            n124 = property on="Tab(Msg/Status)" class="TabCtl (strict)"("Val(Sgnl)"=enum32{"Message", "Status"}."Status" ("Tab(Msg/Status)")) -> ()  [unwired: 2 in, 2 out]
          }
        }
        n125 = local write "MsgString"(w314) -> ()
        n126 = local write "Arguments"(w313) -> ()
        n127 = Search 1D Array(1D array=w311, element=w306) -> (index of element=w309:i32)  [unwired: 1 in]
        n128 = Greater Or Equal To 0?(x=w309) -> (x >= 0?=w308:bool)
        n129 = case shown="True" w308 {
          tunnel: w310 -> [_ w327]
          tunnel: w306 -> [_ w326]
          frame False {
          }
          frame True {
            n130 = property on="Property Node" class="CmbBox"(reference=w327, "Value"=w326) -> ()  [unwired: 1 in, 2 out]
          }
        }
      }
      frame "UI: Refresh History List" {
      }
      frame "CSM: Module List Changed", "UI: Refresh CSM List" {
        n131 = control-ref of="CSM"() -> (w340:refnum<vi>)
        n132 = property on="Property Node" class="CmbBox"(reference=w340) -> (reference out=w332:refnum<vi>, "Value"=w336:string)  [unwired: 1 in, 1 out]
        n133 = call "CSM - List Modules.vi"("Scope (Normal)"="Scope") -> ("error out"=w339:errorcluster, "Module Names"=w334:string[])  [unwired: 9 in]
        n134 = Search 1D Array(1D array=w334, element=w336) -> (index of element=w338:i32)  [unwired: 1 in]
        n135 = Greater Or Equal To 0?(x=w338) -> (x >= 0?=w337:bool)
        n136 = Index Array(array=w334) -> (element=w335:string)  [unwired: 1 in]
        n137 = Select(t=w336, s=w337, f=w335) -> (s? t:f=w333:string)
        n138 = property on="Property Node" class="CmbBox"(reference=w332, "Strings[]"=w334, "Value"=w333) -> ()  [unwired: 1 in, 2 out]
        n139 = call <vilib>:"Simple Error Handler.vi"("error in (no error)"=w339) -> ()  [unwired: 4 in, 5 out]
      }
      frame "UI: Refresh UI" {
      }
      frame "---------- Macro ----------" {
        # "Do not put any code in this frame.\n(It is a separator no-op. You can make a copy of this frame to create a new Macro frame)"
        n140 = call <vilib>:"Add State(s) to Queue__JKI_lib_State_Machine.vi"("State(s) in (\"\")"=w350) -> ("States Out"=w349:string)  [unwired: 14 in]
      }
      frame "Macro: Initialize" {
        # "Initialization Macro\n(This is called once, when the VI starts)"
        n141 = call <vilib>:"Add State(s) to Queue__JKI_lib_State_Machine.vi"("State(s) in Front (\"\")"="Data: Initialize\nData: Initialize References\nInitialize Core Data\nUI: Initialize\nData: Load Arguments Config File\nUI: Front Panel State >> Open\nUI: Refresh CSM List\nUI: Refresh History List\nUI: Refresh UI\nAction: Refresh API List\nAction: Change Btn States", "State(s) in (\"\")"=w355) -> ("States Out"=w354:string)  [unwired: 13 in]
      }
      frame "Macro: Exit" {
        # "Exit Macro\n(This is called once, when the VI exits)"
        n142 = call "FGV-JKISM Modules.vi"("Enum"=_action."Broadcast", "Message"="Macro: Exit") -> ()  [unwired: 8 in, 2 out]
        n143 = call <vilib>:"Add State(s) to Queue__JKI_lib_State_Machine.vi"("State(s) at Back (\"\")"="Data: Save Arguments Config File\nData: Cleanup\nExit") -> ("States Out"=w358:string)  [unwired: 14 in]
        n144 = call <vilib>:"Add State(s) to Queue__JKI_lib_State_Machine.vi"("State(s) in Front (\"\")"=w358, "State(s) in (\"\")"=w363) -> ("States Out"=w362:string)  [unwired: 13 in]
      }
      frame "---------- Action ----------" {
        # "Template Separator\n(You can make a copy of, or modify, this frame)"
        n145 = call <vilib>:"Add State(s) to Queue__JKI_lib_State_Machine.vi"("State(s) in (\"\")"=w367) -> ("States Out"=w366:string)  [unwired: 14 in]
      }
      frame "Action: Send CSM Message" {
        n146 = local read "CSM"() -> (w372:string)
        n147 = Multiply(x=1000, y="Timeout(s)") -> (x*y=w369:i32)
        n148 = case shown="Default" "MsgString" {
          selector: "MsgString" -> [_ w386]
          tunnel: "Arguments" -> [_ w385]
          tunnel: [_ w391] -> w373
          tunnel: w372 -> [_ w384]
          tunnel: [_ w383] -> w371
          tunnel: w369 -> [_ w390]
          frame "" {
          }
          frame Default {
            n149 = call "CSM - Send Message and Wait for Reply.vi"("Response Timeout (-2 Using Global Settings)"=w390, "Current Module (\"\" to Generate an ID)"="Tool-Testpnl" ("Current Module(\"\" to generate an ID)"), "Target Module"=w384, "Arguments (\"\")"=w385, "State"=w386) -> ("error out"=w391:errorcluster, "Response"=w393:string)  [unwired: 4 in, 1 out]
            n150 = call-poly "Build Message with Arguments++.vi"("State With Arguments"=w386, "Arguments (\"\")"=w385, "Target Module (\"\")"=w384) -> ("CSM Message String"=w388:string)  [unwired: 12 in]
            n151 = case shown="True" "Revert Safe String" {
              tunnel: w393 -> [w394 w396]
              tunnel: [w394 w395] -> w380
              frame False {
              }
              frame True {
                n152 = call "CSM - Revert Arguments-Safe String.vi"("Safe Argument String"=w396) -> ("Origin Argument String"=w395:string)  [unwired: 8 in]
              }
            }
            "Response" <- w380
            n153 = call "CSM - Make String Arguments Safe.vi"("Argument String"=w388) -> ("Safe Argument String"=w387:string)  [unwired: 8 in]
            n154 = call <vilib>:"Build State String with Arguments__JKI_lib_State_Machine.vi"("Arguments (\"\")"=w387, "State"="Data: Update Message List" ("State(s) in Front (\"\")")) -> ("State with Arguments"=w382:string)  [unwired: 4 in]
            n155 = call <vilib>:"Add State(s) to Queue__JKI_lib_State_Machine.vi"("State(s) in (\"\")"=w382, "State(s) at Back (\"\")"="UI: Refresh History List\nData: Save Arguments Config File" ("State(s) in Front (\"\")")) -> ("States Out"=w383:string)  [unwired: 13 in]
          }
        }
        n156 = call <vilib>:"Add State(s) to Queue__JKI_lib_State_Machine.vi"("State(s) in (\"\")"=w378, "State(s) at Back (\"\")"=w371) -> ("States Out"=w377:string)  [unwired: 13 in]
      }
      frame "Action: Post CSM Message" {
        # "Your code here.\n(You can make a copy of, or modify, this frame)"
        n157 = local read "MsgString"() -> (w397:string)
        n158 = local read "Arguments"() -> (w398:string)
        n159 = local read "CSM"() -> (w400:string)
        n160 = case shown="Default" w397 {
          selector: w397 -> [_ w410]
          tunnel: w398 -> [_ w409]
          tunnel: [_ w414] -> w401
          tunnel: w400 -> [_ w408]
          tunnel: [_ w407] -> w399
          frame "" {
          }
          frame Default {
            n161 = call "CSM - Post Message.vi"("Current Module (\"\" to Generate an ID)"="Tool-Testpnl" ("Current Module(\"\" to generate an ID)"), "Target Module"=w408, "Arguments (\"\")"=w409, "State"=w410) -> ("error out"=w414:errorcluster)  [unwired: 7 in]
            n162 = call-poly "Build Message with Arguments++.vi"("State With Arguments"=w410, "Arguments (\"\")"=w409, "Target Module (\"\")"=w408) -> ("CSM Message String"=w412:string)  [unwired: 12 in]
            n163 = call "CSM - Make String Arguments Safe.vi"("Argument String"=w412) -> ("Safe Argument String"=w411:string)  [unwired: 8 in]
            n164 = call <vilib>:"Build State String with Arguments__JKI_lib_State_Machine.vi"("Arguments (\"\")"=w411, "State"="Data: Update Message List" ("State(s) in Front (\"\")")) -> ("State with Arguments"=w406:string)  [unwired: 4 in]
            n165 = call <vilib>:"Add State(s) to Queue__JKI_lib_State_Machine.vi"("State(s) in (\"\")"=w406, "State(s) at Back (\"\")"="UI: Refresh History List\nData: Save Arguments Config File" ("State(s) in Front (\"\")")) -> ("States Out"=w407:string)  [unwired: 13 in]
          }
        }
        n166 = call <vilib>:"Add State(s) to Queue__JKI_lib_State_Machine.vi"("State(s) in (\"\")"=w404, "State(s) at Back (\"\")"=w399) -> ("States Out"=w403:string)  [unwired: 13 in]
      }
      frame "Action: Broadcast Status" {
        # "Your code here.\n(You can make a copy of, or modify, this frame)"
        n167 = local read "MsgString"() -> (w416:string)
        n168 = local read "Arguments"() -> (w417:string)
        n169 = local read "CSM"() -> (w419:string)
        n170 = case shown="Default" w416 {
          selector: w416 -> [_ w426]
          tunnel: w417 -> [_ w425]
          tunnel: [_ w427] -> w420
          tunnel: w419 -> [_ w424]
          tunnel: [_ w432] -> w418
          frame "" {
          }
          frame Default {
            (unwired) "Tool-Testpnl" ("Current Module(\"\" to generate an ID)")
            n171 = call "CSM - Request CSM to Broadcast Status Change.vi"("Module Name"=w424, "Arguments (\"\")"=w425, "Status"=w426) -> ("error out"=w427:errorcluster)  [unwired: 8 in]
            n172 = call-poly "Build Message with Arguments++.vi"("State With Arguments"=w426, "Arguments (\"\")"=w425) -> ("CSM Message String"=w434:string)  [unwired: 13 in]
            n173 = Concatenate Strings(w434, "//" ("string"), w424) -> (w429:string)
            n174 = call "CSM - Make String Arguments Safe.vi"("Argument String"=w429) -> ("Safe Argument String"=w433:string)  [unwired: 8 in]
            n175 = call <vilib>:"Build State String with Arguments__JKI_lib_State_Machine.vi"("Arguments (\"\")"=w433, "State"="Data: Update Message List" ("State(s) in Front (\"\")")) -> ("State with Arguments"=w431:string)  [unwired: 4 in]
            n176 = call <vilib>:"Add State(s) to Queue__JKI_lib_State_Machine.vi"("State(s) in (\"\")"=w431, "State(s) at Back (\"\")"="UI: Refresh History List\nData: Save Arguments Config File" ("State(s) in Front (\"\")")) -> ("States Out"=w432:string)  [unwired: 13 in]
          }
        }
        n177 = call <vilib>:"Add State(s) to Queue__JKI_lib_State_Machine.vi"("State(s) in (\"\")"=w423, "State(s) at Back (\"\")"=w418) -> ("States Out"=w422:string)  [unwired: 13 in]
      }
      frame "Action: Change Btn States" {
      }
      frame "Action: Refresh API List" {
        n178 = local read "Tab(Msg/Status)"() -> (w443:enum32{"Message", "Status"})
        n179 = local read "CSM"() -> (w444:string)
        n180 = in-place {
          in-place-border: w444 -> [w455]
          in-place-border: [w454] -> w447
          n181 = in-place-cluster #1(w446) -> ("CSM Check History"=w453:string[])
          n182 = Search 1D Array(1D array=w453, element=w455) -> (index of element=w456:i32)  [unwired: 1 in]
          n183 = Less Than 0?(x=w456) -> (x < 0?=w454:bool)
          n184 = case shown="True" w454 {
            tunnel: w453 -> [w457 w460]
            tunnel: w455 -> [_ w459]
            tunnel: [w457 w458] -> w452
            frame False {
            }
            frame True {
              n185 = Build Array (concatenate)(w460, w459) -> (w458:string[])
            }
          }
          n186 = in-place-cluster #1("CSM Check History"=w452) -> (w445:T8)
        }
        n187 = call "CSM - Check If Module Exists.vi"("CSM Name"=w444) -> ("error out"=w440:errorcluster, "Exist?"=w441:bool, "CSM Name (Dup)"=w450:string)  [unwired: 8 in]
        n188 = Not(x=w440) -> (.not. x?=w439:bool)
        n189 = And(x=w441, y=w439) -> (x .and. y?=w442:bool)
        n190 = case shown="True" w442 {
          tunnel: w450 -> [_ w477]
          tunnel: w449 -> [_ w476]
          tunnel: [_ w478] -> w448
          tunnel: w447 -> [_ w475]
          tunnel: w443 -> [w461 w474]
          frame False {
            n191 = case shown="\"Message\", Default" w461 {
              tunnel: [T6."Enabled" ("Disabled") T6."Disabled and Grayed Out" ("Disabled")] -> w462
              frame "Message", Default {
              }
              frame "Status" {
              }
            }
            n192 = property on="Revert Safe String" class="Bool (strict)"("DisabledEnum"=w462) -> ()  [unwired: 2 in, 2 out]
            n193 = property on="Arguments" class="Str"("DisabledEnum"=w462) -> ()  [unwired: 2 in, 2 out]
            n194 = property on="Response" class="Str"("DisabledEnum"=w462) -> ()  [unwired: 2 in, 2 out]
          }
          frame True {
            n195 = case shown="\"Message\"" w474 {
              tunnel: [w484 w498] -> w478
              tunnel: w477 -> [w486 w497]
              tunnel: w476 -> [w485 w496]
              tunnel: w475 -> [w483 w495]
              tunnel: [w480 w493] -> w471
              tunnel: [T6."Disabled and Grayed Out" ("Disabled") T6."Enabled" ("Disabled")] -> w469
              frame "Status" {
                n196 = call "Read CSM Status with lvcsm Support.vi"("Current Module (\"\" to Generate an ID)"=w485, "Force? (F)"=w483, "CSM Name"=w486) -> ("error out"=w484:errorcluster, "CSMAPI List"=w482:string[])  [unwired: 7 in]
                n197 = for {
                  tunnel: w482 -> [w490] mode=indexing
                  tunnel: [w487] -> w481 mode=indexing
                  n198 = Match Pattern(string=w490, regular expression="@") -> (before substring=w488:string)  [unwired: 1 in, 3 out]
                  n199 = call "Trim Single-line Text.vi"("single-line text"=w488) -> ("trimed text"=w487:string)  [unwired: 2 in]
                }
                n200 = call "Remove Duplicates From StrArray.vi"("StrArray In"=w481) -> ("StrArray"=w480:string[])  [unwired: 9 in, 1 out]
              }
              frame "Message" {
                n201 = call "Read CSM States with lvcsm Support.vi"("Current Module (\"\" to Generate an ID)"=w496, "Force? (F)"=w495, "CSM Name"=w497) -> ("error out"=w498:errorcluster, "CSMAPI List"=w494:string[])  [unwired: 7 in]
                n202 = call "filter CSM States.vi"("Interface-Filter"="Interface-Filter", "Array"=w494) -> ("filtered array"=w493:string[])  [unwired: 9 in]
              }
            }
            n203 = property on="Revert Safe String" class="Bool (strict)"("DisabledEnum"=w469) -> ()  [unwired: 2 in, 2 out]
            n204 = property on="Arguments" class="Str"("DisabledEnum"=w469) -> ()  [unwired: 2 in, 2 out]
            n205 = property on="Response" class="Str"("DisabledEnum"=w469) -> ()  [unwired: 2 in, 2 out]
            n206 = property on="Message/Status" class="CmbBox"("Strings[]"=w471) -> ("Value"=w472:string)  [unwired: 2 in, 2 out]
            n207 = Search 1D Array(1D array=w471, element=w472) -> (index of element=w473:i32)  [unwired: 1 in]
            n208 = Index Array(array=w471) -> (element=w466:string)  [unwired: 1 in]
            n209 = Greater Or Equal To 0?(x=w473) -> (x >= 0?=w467:bool)
            n210 = Empty String/Path?(string/path=w466) -> (empty?=w465:bool)
            n211 = Or(x=w467, y=w465) -> (x .or. y?=w468:bool)
            n212 = Select(t=w472, s=w468, f=w466) -> (s? t:f=w470:string)
            n213 = property on="Message/Status" class="CmbBox"("Value"=w470) -> ()  [unwired: 2 in, 2 out]
          }
        }
      }
      frame "No Peroidic Log over 1s" {
        n214 = call "CSM - Generate User Global Log.vi"("Place (\"\" to Use VI's Name)"=w499, "Log"="No Peroidic Log over 1s.") -> ()  [unwired: 9 in, 1 out]
      }
    }
  }
  n215 = disable-structure shown="Disabled" {
    frame Disabled {
      n216 = case shown="\"Module Created\", \"Module Destroyed\"" {
        selector: _ -> [_ _]
        tunnel: _ -> [_ w505]
        frame "User Log", Default {
        }
        frame "Module Created", "Module Destroyed" {
          n217 = Generate User Event(user event=w505, event data cluster="UI: Refresh CSM List" ("State(s) in Front (\"\")")) -> ()  [unwired: 2 in, 2 out]
        }
      }
    }
    frame Enabled {
    }
  }
  n218 = control-ref of="Current VI Reference"() -> (w3:refnum<vi>)
  n219 = call "Close FP if in LabVIEW Dir.vi"("VI Refnum"=w3, "Error in"=w2) -> ("Error out"=w4:errorcluster)  [unwired: 9 in]
  n220 = call <vilib>:"Clear Errors.vi"("error in (no error)"=w4) -> ()  [unwired: 5 in, 2 out]
